vi "dfd_Compute Coefficients of QMF Lattice.vi"(8 "error in (no error)":errorcluster, 10 "F 0":dbl[](array[numeric]), 11 "H 0":dbl[](array[numeric])) -> (0 "error":errorcluster, 2 "k":dbl[](array[numeric]))   [LabVIEW 2017, in "NI_DigFilter_FilterBank.lvlib"]
doc: "Computes the lattice coefficients of the QMF filter bank from its prototype filter coefficients."
uses:
  <vilib>/addons/Digital Filter Design/NI_DigFilter_FilterBank.lvlib
  <vilib>/addons/Digital Filter Design/NI_DigFilterLicensed.lvlib
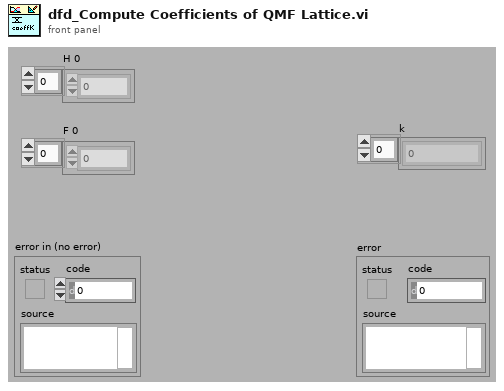
[diagram p1: front panel]
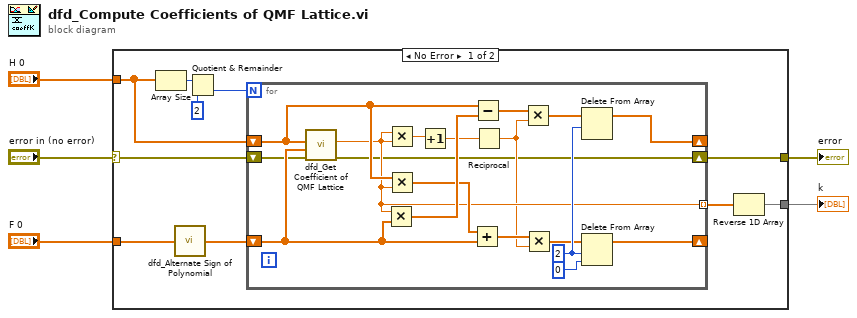
[diagram p0: block diagram]
diagram:
  n1 = case shown="No Error" "error in (no error)" {
    selector: "error in (no error)" -> [w8 w34]
    tunnel: [w13 _] -> w3
    tunnel: [w10 w34] -> w4
    tunnel: "H 0" -> [w9 _]
    tunnel: "F 0" -> [w7 _]
    frame No Error {
      n2 = Array Size(array=w9) -> (size(s)=w12:i32)
      n3 = call <vilib>:"dfd_Alternate Sign of Polynomial.vi"("polynomial in"=w7) -> ("polynomial out"=w6:dbl[])  [unwired: 1 in]
      n4 = Quotient & Remainder(x=w12, y=2) -> (floor(x/y)=w11:i32)  [unwired: 1 out]
      n5 = for {
        N: w11 -> [_]
        shift-right: [w28] -> _
        shift-left: w9 -> [w20]
        shift-right: [w31] -> _
        shift-left: w6 -> [w26]
        tunnel: [w19] -> w14 mode=indexing
        shift-right: [w16] -> w10
        shift-left: w8 -> [w17]
        w29 = 2
        n6 = call <vilib>:"dfd_Get Coefficient of QMF Lattice.vi"("error in (no error)"=w17, "hm1"=w26, "hm0"=w20) -> ("error out"=w16:errorcluster, "am"=w19:dbl)  [unwired: 7 in]
        n7 = Multiply(x=w19, y=w26) -> (x*y=w32:dbl[])
        n8 = Multiply(x=w19, y=w19) -> (x*y=w33:dbl)
        n9 = Multiply(x=w20, y=w19) -> (x*y=w25:dbl[])
        n10 = Increment(x=w33) -> (x+1=w27:dbl)
        n11 = Add(x=w25, y=w26) -> (x+y=w23:dbl[])
        n12 = Subtract(x=w20, y=w32) -> (x-y=w24:dbl[])
        n13 = Reciprocal(x=w27) -> (1/x=w18:dbl)
        n14 = Multiply(x=w24, y=w18) -> (x*y=w22:dbl[])
        n15 = Multiply(x=w23, y=w18) -> (x*y=w21:dbl[])
        n16 = Delete From Array(array=w22, length=w29) -> (array with subset deleted=w28:dbl[])  [unwired: 1 in, 1 out]
        n17 = Delete From Array(array=w21, length=w29, index=0) -> (array with subset deleted=w31:dbl[])  [unwired: 1 out]
      }
      n18 = Reverse 1D Array(array=w14) -> (reversed array=w13:dbl[])
    }
    frame Error {
    }
  }
  "k" <- w3
  "error" <- w4
